vi "Switch Append Group Data Fields.vi"(10 "Switch Results":T1, 11 "Fields In":T3[](array[typedef])) -> (3 "Fields Out":T3[](array[typedef]))   [LabVIEW 2011]
uses:
  server/database/Fields/Field Record.ctl
  server/database/Fields/Field DataTypes.ctl
  server/database/Fields/Field NextItem.ctl
  TypeDefs/Switch Results.ctl
  server/database/Stations/Instruments/Instrument Record.ctl
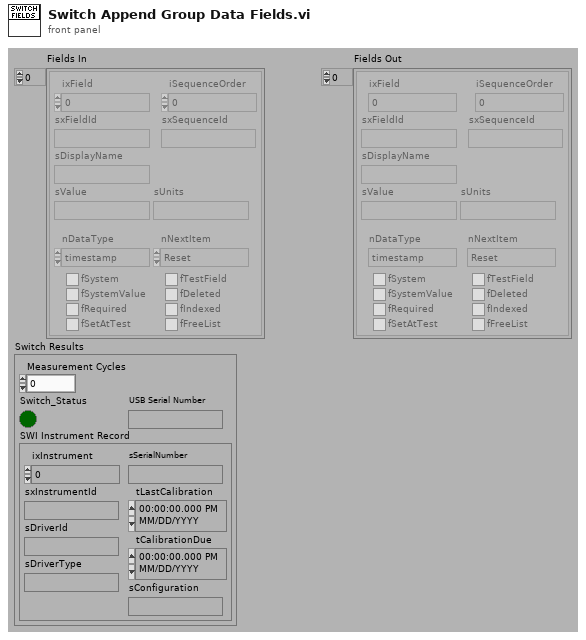
[diagram p1: front panel]
types:
  T1 = typedef "Switch Results.ctl" = cluster{"Measurement Cycles":i32, "Switch_Status":bool, "USB Serial Number":string, "SWI Instrument Record":T2}
  T2 = typedef "Instrument Record.ctl" = cluster{"ixInstrument":i32, "sxInstrumentId":string, "sDriverId":string, "sDriverType":string, "sSerialNumber":string, "tLastCalibration":timestamp, "tCalibrationDue":timestamp, "sConfiguration":string}
  T3 = typedef "Field Record.ctl" = cluster{"ixField":i32, "iSequenceOrder":i32, "sxFieldId":string, "sxSequenceId":string, "sDisplayName":string, "sValue":string, "sUnits":string, "nDataType":T4, "nNextItem":T5, "fSystem":bool, "fSystemValue":bool, "fRequired":bool, "fSetAtTest":bool, "fTestField":bool, "fDeleted":bool, "fIndexed":bool, "fFreeList":bool}
  T4 = typedef "Field DataTypes.ctl" = enum32{"text", "numeric", "list", "timestamp", "boolean"}
  T5 = typedef "Field NextItem.ctl" = enum32{"Reset", "Retain", "Auto-Increment"}
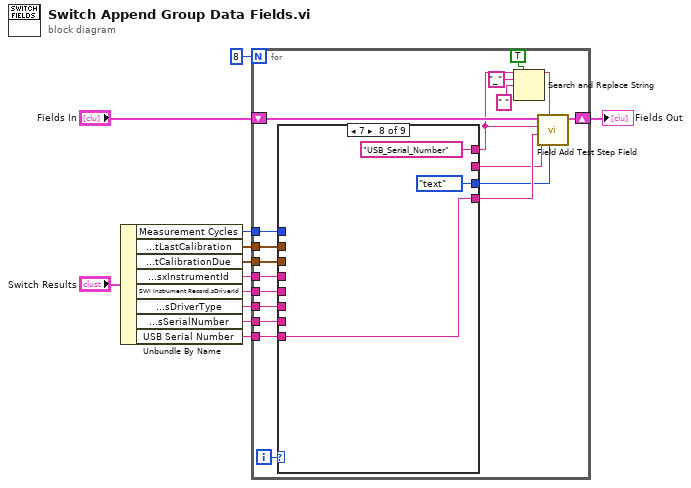
[diagram p0: block diagram]
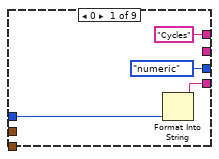
[diagram p2: hidden frame]
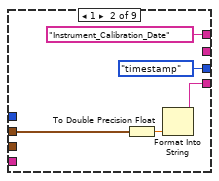
[diagram p3: hidden frame]
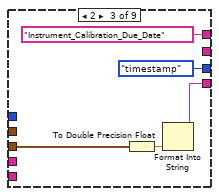
[diagram p4: hidden frame]
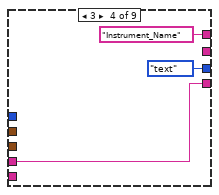
[diagram p5: hidden frame]
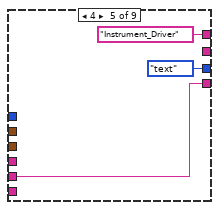
[diagram p6: hidden frame]
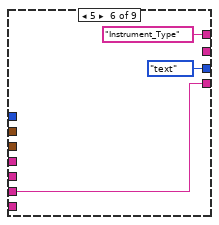
[diagram p7: hidden frame]
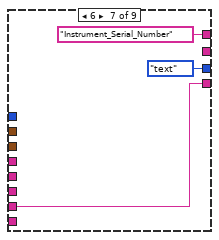
[diagram p8: hidden frame]
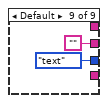
[diagram p9: hidden frame]
diagram:
  n1 = Unbundle By Name("Switch Results") -> ("Measurement Cycles"=w8:i32, "SWI Instrument Record.tLastCalibration"=w7:timestamp, "SWI Instrument Record.tCalibrationDue"=w6:timestamp, "SWI Instrument Record.sxInstrumentId"=w5:string, "SWI Instrument Record.sDriverId"=w4:string, "SWI Instrument Record.sDriverType"=w3:string, "SWI Instrument Record.sSerialNumber"=w2:string, "USB Serial Number"=w1:string)
  n2 = for {
    N: 8 -> [_]
    tunnel: w8 -> [w30]
    shift-right: [w28] -> w11
    shift-left: "Fields In" -> [w29]
    tunnel: w7 -> [w24]
    tunnel: w6 -> [w23]
    tunnel: w5 -> [w22]
    tunnel: w4 -> [w21]
    tunnel: w3 -> [w20]
    tunnel: w2 -> [w19]
    tunnel: w1 -> [w13]
    i -> [w31]
    n3 = case shown="7" w31 {
      tunnel: w30 -> [w33 _ _ _ _ _ _ _ _]
      tunnel: ["Cycles" ("Field_ID") "Instrument_Calibration_Date" ("Field_ID") "Instrument_Calibration_Due_Date" ("Field_ID") "Instrument_Name" ("Field_ID") "Instrument_Driver" ("Field_ID") "Instrument_Type" ("Field_ID") "Instrument_Serial_Number" ("Field_ID") "USB_Serial_Number" ("Field_ID") _] -> w15
      tunnel: [Field_DataTypes."numeric" ("Data Type") Field_DataTypes."timestamp" ("Data Type") Field_DataTypes."timestamp" ("Data Type") Field_DataTypes."text" ("Data Type") Field_DataTypes."text" ("Data Type") Field_DataTypes."text" ("Data Type") Field_DataTypes."text" ("Data Type") Field_DataTypes."text" ("Data Type") Field_DataTypes."text" ("Data Type")] -> w26
      tunnel: [w34 w37 w42 w46 w49 w52 w55 w58 _] -> w27
      tunnel: [_ _ _ _ _ _ _ _ ""] -> w25
      tunnel: w24 -> [_ w36 _ _ _ _ _ _ _]
      tunnel: w23 -> [_ _ w41 _ _ _ _ _ _]
      tunnel: w22 -> [_ _ _ w46 _ _ _ _ _]
      tunnel: w21 -> [_ _ _ _ w49 _ _ _ _]
      tunnel: w20 -> [_ _ _ _ _ w52 _ _ _]
      tunnel: w19 -> [_ _ _ _ _ _ w55 _ _]
      tunnel: w13 -> [_ _ _ _ _ _ _ w58 _]
      frame 0 {
        n4 = Format Into String(w33) -> (resulting string=w34:string)  [unwired: 3 in, 1 out]
      }
      frame 1 {
        n5 = To Double Precision Float(number=w36) -> (double precision float=w38:dbl)
        n6 = Format Into String(w38) -> (resulting string=w37:string)  [unwired: 3 in, 1 out]
      }
      frame 2 {
        n7 = To Double Precision Float(number=w41) -> (double precision float=w43:dbl)
        n8 = Format Into String(w43) -> (resulting string=w42:string)  [unwired: 3 in, 1 out]
      }
      frame 3 {
      }
      frame 4 {
      }
      frame 5 {
      }
      frame 6 {
      }
      frame 7 {
      }
      frame Default {
      }
    }
    n9 = Search and Replace String(replace all?=TRUE ("replace all? (F)"), input string=w15, search string="_", replace string=" " ("replace string (\"\")")) -> (result string=w14:string)  [unwired: 1 in, 6 out]
    n10 = call "Field Add Test Step Field.vi"("nDataType"=w26, "sDisplayName"=w14, "sUnits"=w25, "sValue"=w27, "sxFieldId"=w15, "Fields In"=w29) -> ("Fields Out"=w28:T3[])  [unwired: 5 out]
  }
  "Fields Out" <- w11
